vi "VISA Test.vi"(8 "error in":errorcluster, 11 "VISA resource name":refnum<visa-resource-name>) -> (0 "error out":errorcluster, 3 "VISA resource name out":refnum<visa-resource-name>)   [LabVIEW 2020, in "ChromTech Series III Pump.lvlib"]
doc: "Simple VI designed to test VISA communication to the instrument. This application opens a session to the instrument, performs a write of the fetch ID command \"ID\\r\", and queries the device for its response."
uses:
  ChromTech Series III Pump.lvlib
panel:
  out "Instrument Response":string
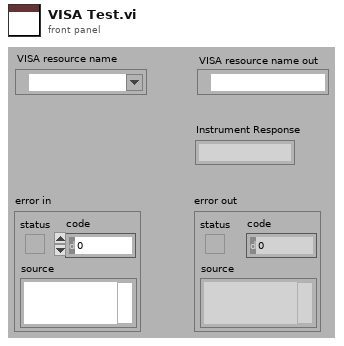
[diagram p1: front panel]
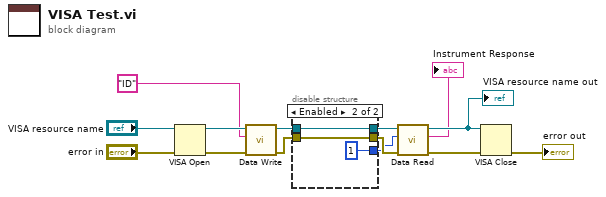
[diagram p0: block diagram]
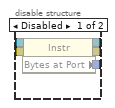
[diagram p2: hidden frame]
diagram:
  n1 = VISA Open(error in (no error)="error in", VISA resource name="VISA resource name") -> (VISA resource name=w12:refnum<visa-resource-name>, error out=w11:errorcluster)  [unwired: 3 in]
  n2 = call "Data Write.vi"("error in (no error)"=w11, "Command"="ID", "VISA Refnum in"=w12) -> ("error out"=w3:errorcluster, "VISA Refnum out"=w5:refnum<visa-resource-name>)  [unwired: 7 in]
  n3 = disable-structure shown="Enabled" {
    disable-tunnel: w5 -> [w19 w22]
    disable-tunnel: [w18 w22] -> w4
    disable-tunnel: w3 -> [w17 w21]
    disable-tunnel: [w16 w21] -> w2
    disable-tunnel: [w15 1] -> w1
    frame Disabled {
      n4 = property class="Instr"(reference=w19, error in=w17) -> (reference out=w18:refnum<visa-resource-name>, error out=w16:errorcluster, "Bytes at Port"=w15:u32)
    }
    frame Enabled {
    }
  }
  n5 = call "Data Read.vi"("error in (no error)"=w2, "Bytes to read"=w1, "VISA Refnum in"=w4) -> ("error out"=w10:errorcluster, "read buffer"=→"Instrument Response":string, "VISA Refnum out"=w8:refnum<visa-resource-name>)  [unwired: 6 in]
  "VISA resource name out" <- w8
  n6 = VISA Close(VISA resource name=w8, error in (no error)=w10) -> (error out=→"error out":errorcluster)
